vi "Autosize MCListbox Columns.vi"(4 "error in (no error)":errorcluster, 6 "Options":T1={"Whitespace Border"=10, "Resize Table"=FALSE, "Number of Columns"=20, "Default Width"=50}, 7 "Multicolumn Ref":refnum<vi>) -> (0 "error out":errorcluster)   [LabVIEW 2015]
doc: "This VI resizes each column of the table specified by Table Ref based on the widest entry of the column. Additionally, if Resize Table? is TRUE, the VI will set the table width based on the number of populated columns."
panel:
  # "The original code was found in NI Discussion Forum, by ceger\nhttp://forums.ni.com/ni/board/message?board.id=170&message.id=356189\n\nThis version is modified to handle\n1)\tRow's Header column and added default width size for empty table.\n2)\tRun from JKI right-click framework\n3)\tChanged control type to MultiColumnListBox."
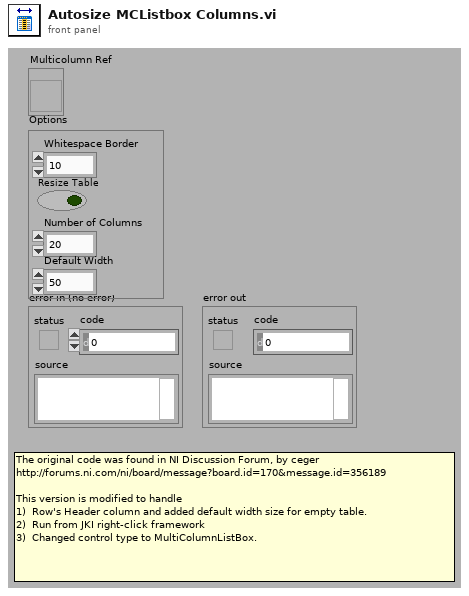
[diagram p1: front panel]
types:
  T1 = cluster{"Whitespace Border":i16, "Resize Table":bool, "Number of Columns":i32, "Default Width":u32}
  T2 = enum16{"User-specified Font", "Application Font", "System Font", "Dialog Font"}
  T3 = cluster{"Font Name:":string, "Size":i16, "Strikeout?":bool, "Italic?":bool, "Underline?":bool, "Outline?":bool, "Shadow?":bool, "Bold?":bool}
  T4 = typedef "LVRowAndColumnTypeDef.ctl" = cluster{"Row":i32, "Column":i32}
  T5 = cluster{"left":i16, "top":i16, "right":i16, "bottom":i16}
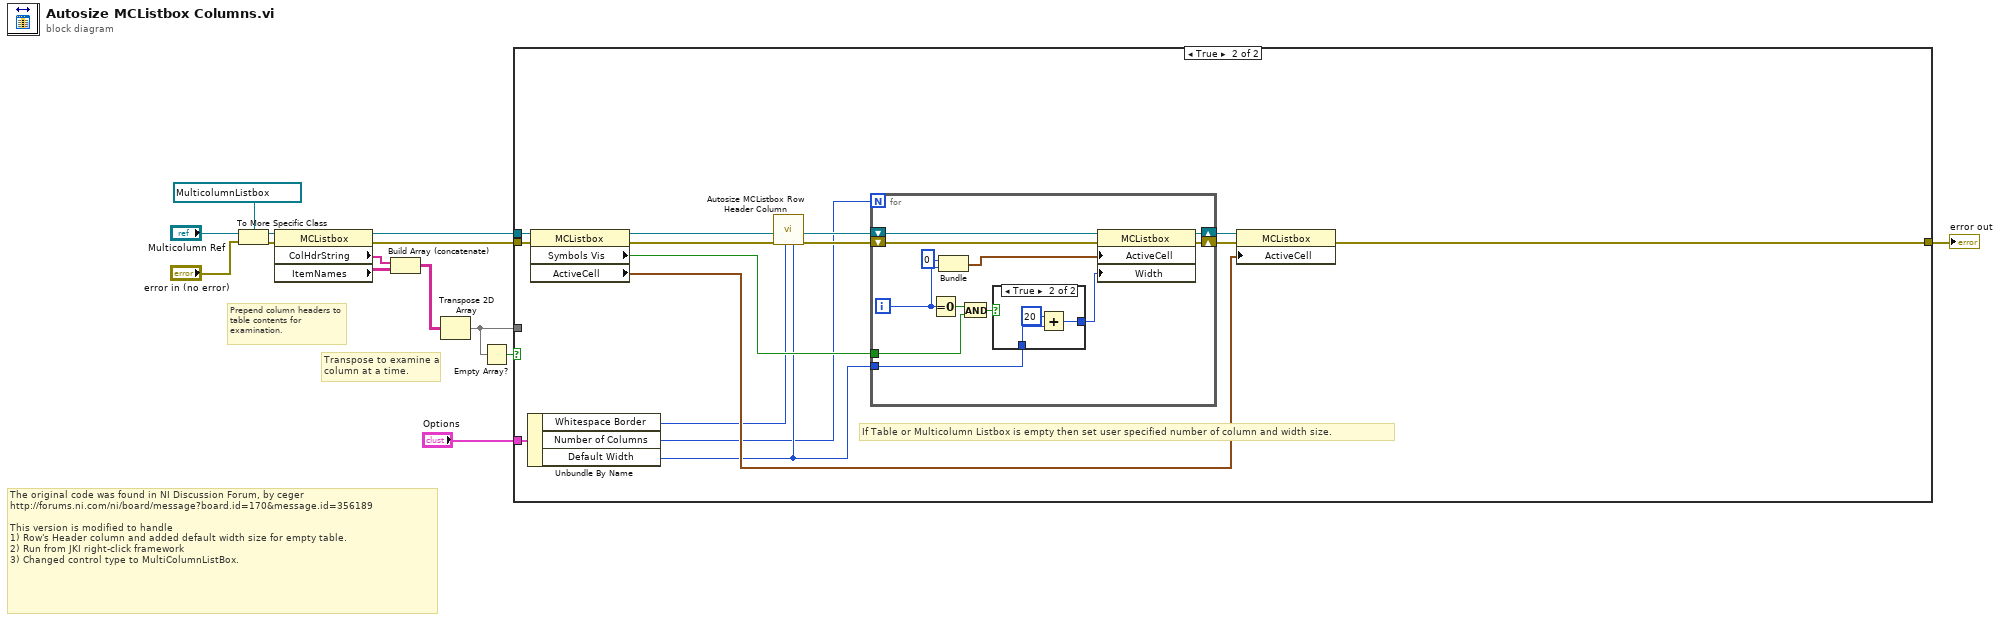
[diagram p0: block diagram]
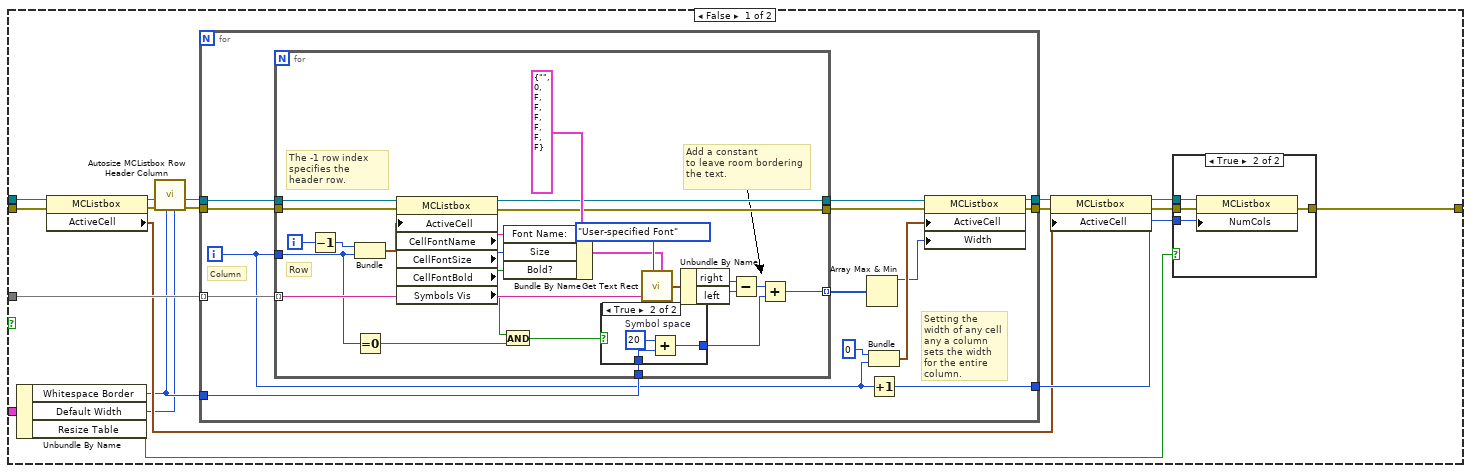
[diagram p2: hidden frame]
diagram:
  # "The original code was found in NI Discussion Forum, by ceger\nhttp://forums.ni.com/ni/board/message?board.id=170&message.id=356189\n\nThis version is modified to handle\n1)\tRow's Header column and added default width size for empty table.\n2)\tRun from JKI right-click framework\n3)\tChanged control type to MultiColumnListBox."
  # "Transpose to examine a column at a time."
  # "Prepend column headers to table contents for examination."
  n1 = To More Specific Class(target class=refnum<vi> refnum ("Multicolumn Listbox"), reference="Multicolumn Ref", error in="error in (no error)") -> (specific class reference=w8:refnum<vi>, error out=w6:errorcluster)
  n2 = property class="MCListbox"(reference=w8, error in=w6) -> (reference out=w14:refnum<vi>, error out=w12:errorcluster, "ColHdrString"=w2:string[], "ItemNames"=w11:string[][])
  n3 = Build Array (concatenate)(w2, w11) -> (w13:string[][])
  n4 = Transpose 2D Array(2D array=w13) -> (transposed array=w1:string[][])
  n5 = Empty Array?(array=w1) -> (empty?=w4:bool)
  n6 = case shown="True" w4 {
    tunnel: w14 -> [w24 w94]
    tunnel: w12 -> [w25 w95]
    tunnel: [w31 w92] -> w10
    tunnel: w1 -> [w30 _]
    tunnel: "Options" -> [w22 w89]
    frame False {
      n7 = Unbundle By Name(w22) -> ("Whitespace Border"=w17:i16, "Default Width"=w15:u32, "Resize Table"=w16:bool)
      n8 = property class="MCListbox"(reference=w24, error in=w25) -> (reference out=w20:refnum<vi>, error out=w21:errorcluster, "ActiveCell"=w23:T4)
      n9 = call "Autosize MCListbox Row Header Column.vi"("Default Width"=w15, "Whitespace Border"=w17, "error in"=w21, "reference in"=w20) -> ("error out"=w18:errorcluster, "reference out"=w19:refnum<vi>)  [unwired: 6 out]
      n10 = for {
        tunnel: w30 -> [w51] mode=indexing
        tunnel: w19 -> [w50]
        tunnel: w18 -> [w48]
        tunnel: [w42] -> w29
        tunnel: [w41] -> w27
        tunnel: [w40] -> w32
        tunnel: w17 -> [w39]
        i -> [w38]
        # "Setting the width of any cell any a column sets the width for the entire column."
        # "Column"
        n11 = for {
          tunnel: w51 -> [w69] mode=indexing
          tunnel: w50 -> [w76]
          tunnel: w38 -> [w57]
          tunnel: [w59] -> w49 mode=indexing
          tunnel: w48 -> [w64]
          tunnel: [w63] -> w46
          tunnel: [w62] -> w47
          tunnel: w39 -> [w53]
          i -> [w58]
          # "The -1 row index specifies the header row."
          # "Add a constant\nto leave room bordering the text."
          # "Row"
          n12 = Decrement(x=w58) -> (x-1=w65:i32)
          n13 = Bundle(w65, w57) -> (w75:cluster{i32, i32})  [unwired: 1 out]
          n14 = Equal To 0?(x=w57) -> (x = 0?=w55:bool)
          n15 = property class="MCListbox"(reference=w76, error in=w64, "ActiveCell"=w75) -> (reference out=w62:refnum<vi>, error out=w63:errorcluster, "CellFontName"=w73:string, "CellFontSize"=w60:u32, "CellFontBold"=w72:bool, "Symbols Vis"=w56:bool)
          n16 = And(x=w56, y=w55) -> (x .and. y?=w54:bool)
          n17 = Bundle By Name(cluster=T3 {"Font Name:"="", "Size"=0, "Strikeout?"=FALSE, "Italic?"=FALSE, "Underline?"=FALSE, "Outline?"=FALSE, "Shadow?"=FALSE, "Bold?"=FALSE} ("[user-specified font]"), "Font Name:"=w73, "Size"=w60, "Bold?"=w72) -> (w70:T3)
          n18 = case shown="True" w54 {
            tunnel: w53 -> [w77 w80]
            tunnel: [w77 w79] -> w52
            frame False {
            }
            frame True {
              w78 = i16 20  # Symbol space
              n19 = Add(x=w78, y=w80) -> (x+y=w79:i16)
            }
          }
          n20 = call <vilib>:"Get Text Rect.vi"("desired font(Application)"=T2."User-specified Font", "text"=w69, "[user-specified font]"=w70) -> ("rect"=w68:T5)  [unwired: 3 in, 3 out]
          n21 = Unbundle By Name(w68) -> ("right"=w67:i16, "left"=w66:i16)
          n22 = Subtract(x=w67, y=w66) -> (x-y=w61:i16)
          n23 = Add(x=w61, y=w52) -> (x+y=w59:i16)
        }
        n24 = Array Max & Min(array=w49) -> (max value=w43:i16)  [unwired: 3 out]
        n25 = Bundle(0, w38) -> (w44:cluster{i32, i32})  [unwired: 1 out]
        n26 = Increment(x=w38) -> (x+1=w40:i32)
        n27 = property class="MCListbox"(reference=w47, error in=w46, "ActiveCell"=w44, "Width"=w43) -> (reference out=w41:refnum<vi>, error out=w42:errorcluster)
      }
      n28 = property class="MCListbox"(reference=w27, error in=w29, "ActiveCell"=w23) -> (reference out=w28:refnum<vi>, error out=w26:errorcluster)
      n29 = case shown="True" w16 {
        tunnel: w28 -> [_ w37]
        tunnel: w26 -> [w33 w36]
        tunnel: w32 -> [_ w35]
        tunnel: [w33 w34] -> w31
        frame False {
        }
        frame True {
          n30 = property class="MCListbox"(reference=w37, error in=w36, "NumCols"=w35) -> (error out=w34:errorcluster)  [unwired: 1 out]
        }
      }
    }
    frame True {
      # "If Table or Multicolumn Listbox is empty then set user specified number of column and width size."
      n31 = Unbundle By Name(w89) -> ("Whitespace Border"=w85:i16, "Number of Columns"=w81:i32, "Default Width"=w84:u32)
      n32 = property class="MCListbox"(reference=w94, error in=w95) -> (reference out=w87:refnum<vi>, error out=w86:errorcluster, "Symbols Vis"=w93:bool, "ActiveCell"=w90:T4)
      n33 = call "Autosize MCListbox Row Header Column.vi"("Default Width"=w84, "Whitespace Border"=w85, "error in"=w86, "reference in"=w87) -> ("error out"=w82:errorcluster, "reference out"=w83:refnum<vi>)  [unwired: 6 out]
      n34 = for {
        N: w81 -> [_]
        tunnel: w93 -> [w104]
        shift-right: [w100] -> w91
        shift-left: w83 -> [w101]
        tunnel: w84 -> [w99]
        shift-right: [w97] -> w88
        shift-left: w82 -> [w98]
        i -> [w96]
        n35 = Equal To 0?(x=w96) -> (x = 0?=w105:bool)
        n36 = Bundle(0, w96) -> (w106:cluster{i32, i32})  [unwired: 1 out]
        n37 = And(x=w105, y=w104) -> (x .and. y?=w103:bool)
        n38 = case shown="True" w103 {
          tunnel: w99 -> [w108 w111]
          tunnel: [w108 w109] -> w102
          frame False {
          }
          frame True {
            n39 = Add(x=u32 20, y=w111) -> (x+y=w109:u32)
          }
        }
        n40 = property class="MCListbox"(reference=w101, error in=w98, "ActiveCell"=w106, "Width"=w102) -> (reference out=w100:refnum<vi>, error out=w97:errorcluster)
      }
      n41 = property class="MCListbox"(reference=w91, error in=w88, "ActiveCell"=w90) -> (error out=w92:errorcluster)  [unwired: 1 out]
    }
  }
  "error out" <- w10
